vi "File Exist.vi"(8 "error in (no error)":errorcluster caption="错误输入（无错误）", 10 "Path":path, 11 "FileSystem 输入":refnum<class "FileSystem.lvclass"> caption="DNL_LabVIEW Object in") -> (0 "error out":errorcluster caption="错误输出", 2 "FileExists":bool, 3 "FileSystem 输出":refnum<class "FileSystem.lvclass"> caption="DNL_LabVIEW Object out")   [LabVIEW 2012, in "FileSystem.lvclass"]
uses:
  FileSystem.lvclass
  FileSystem.lvclass/FileSystem.ctl
  Microsoft.VisualBasic
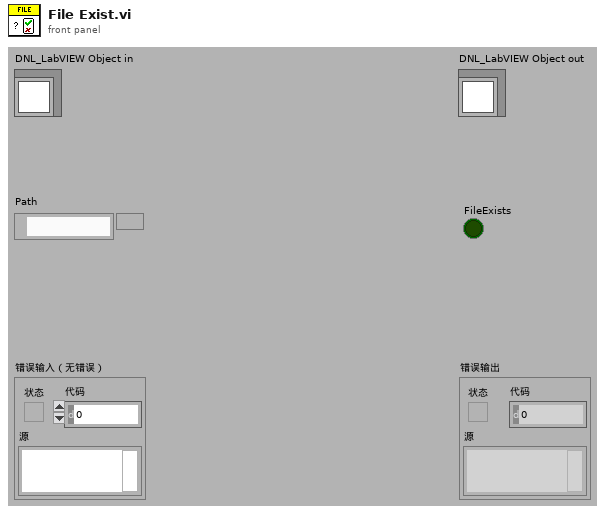
[diagram p1: front panel]
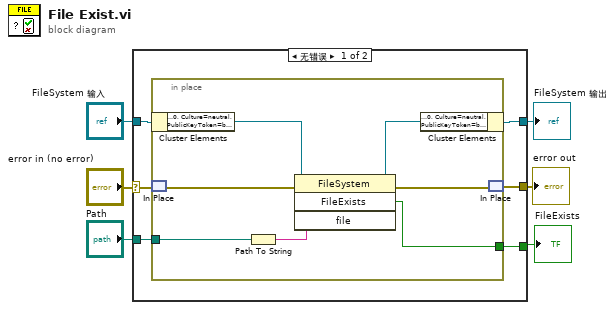
[diagram p0: block diagram]
diagram:
  n1 = case shown="无错误" "error in (no error)" {
    selector: "error in (no error)" -> [w11 w21]
    tunnel: [w10 w21] -> w5
    tunnel: [w9 w20] -> w3
    tunnel: "FileSystem 输入" -> [w12 w20]
    tunnel: "Path" -> [w8 _]
    tunnel: [w7 _] -> w1
    frame No Error {
      n2 = in-place {
        in-place-border: w8 -> [w15]
        in-place-border: [w13] -> w7
        n3 = in-place-cluster #1(w12) -> ("FileSystem"=w19:refnum<k24>)
        n4 = in-place-match #2(w11) -> (w17:errorcluster)
        n5 = Path To String(path=w15) -> (string=w14:string)
        n6 = invoke class="FileSystem" method="FileExists"(reference=w19, error in=w17, "file"=w14) -> (reference out=w18:refnum<k24>, error out=w16:errorcluster, "FileExists"=w13:bool)  [unwired: 1 in, 1 out]
        n7 = in-place-cluster #1("FileSystem"=w18) -> (w9:refnum<class "FileSystem.lvclass">)
        n8 = in-place-match #2(w16) -> (w10:errorcluster)
      }
    }
    frame Error {
    }
  }
  "error out" <- w5
  "FileSystem 输出" <- w3
  "FileExists" <- w1
